vi "_iWorx - Pulse.vi"() -> ()   [LabVIEW 2012]
uses:
  <vilib>/DAQmx/create/channels.llb/DAQmx Create Channel (AI-Voltage-Basic).vi
  <vilib>/DAQmx/configure/timing.llb/DAQmx Timing (Sample Clock).vi
  <vilib>/DAQmx/read.llb/DAQmx Read (Analog 1D Wfm NChan NSamp).vi
  <vilib>/measure/macond.llb/IIR Filter for 1 Chan.vi
  <vilib>/measure/NI_MAPro.lvlib
panel:
  in  "Stop":bool
  in  "Reset Scale":bool
  in  "Log Info Button":bool
  out "Heart Signal":waveform(dbl)(graph)
  out "Avg Pulse":dbl format="%5.1f BPM"
  out "Inst Pulse":dbl format="%5.1f BPM"
  in  "Threshold":dbl=0.0005 step=0.0001 format="%_3p"
  in  "Calibrate":bool
  out "error out":errorcluster
  in  "Set Up":bool
  in  "Channel":u16(ring) items=["Channel 1", "Channel 2"]
  in  "Pause Button":bool
  in  "Snapshot":bool
  in  "Clear Chart":bool
  in  "Open Log":bool
  in  "Rescale Y":bool
  out "Raw Signal":dbl(knob) scale=-1.0..1.0
  # "iWorx - Pulse - Data Logger"
  # "Sensor Input"
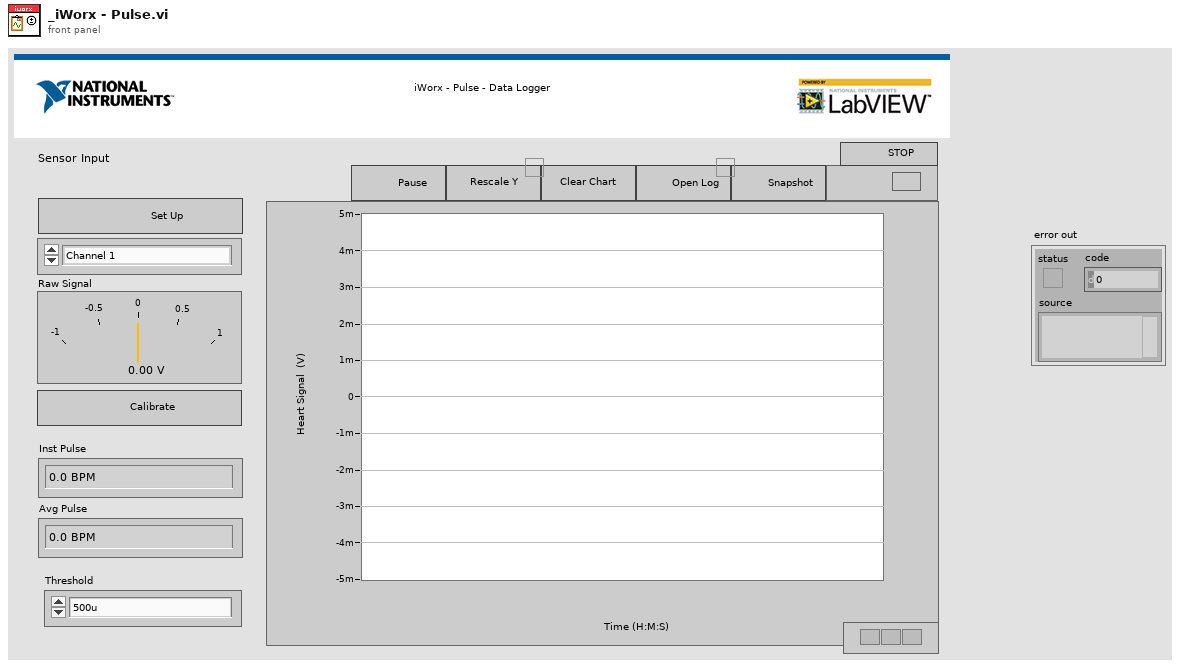
[diagram p1: front panel]
types:
  T1 = cluster{"Topology":enum16{"Off", "Butterworth", "Chebyshev", "Inverse Chebyshev", "Elliptic", "Bessel"}, "Type":enum16{"Lowpass", "Highpass", "Bandpass", "Bandstop"}, "Order":i32, "Lower Fc":dbl, "Upper Fc":dbl, "PB Ripple":dbl, "SB Attenuation":dbl}
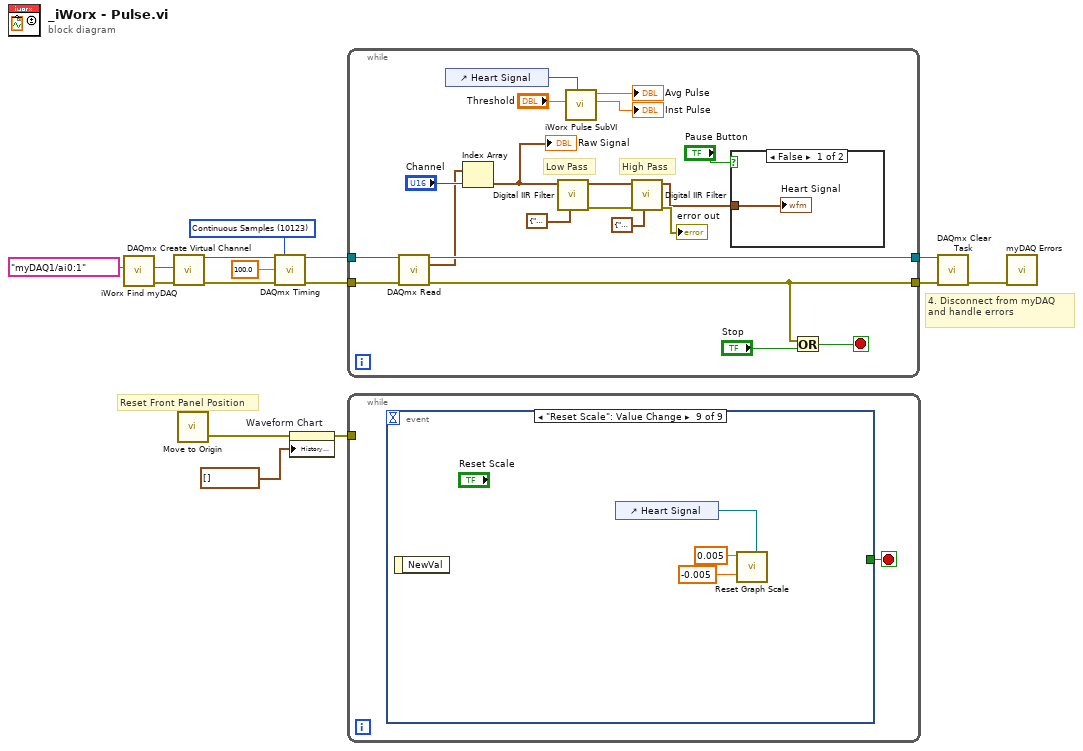
[diagram p0: block diagram]
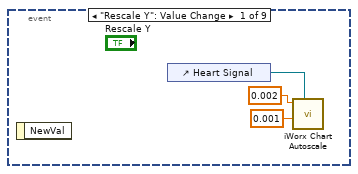
[diagram p2: hidden frame]
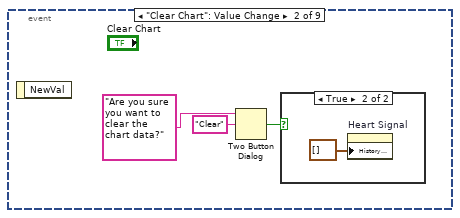
[diagram p3: hidden frame]
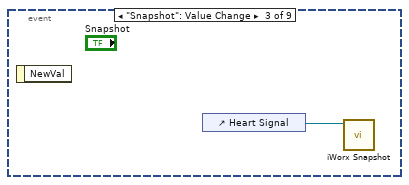
[diagram p5: hidden frame]
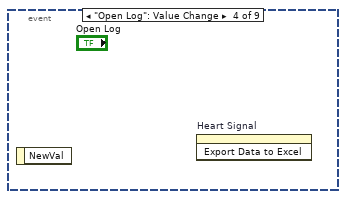
[diagram p6: hidden frame]
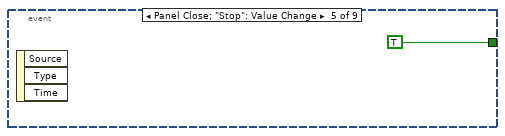
[diagram p7: hidden frame]
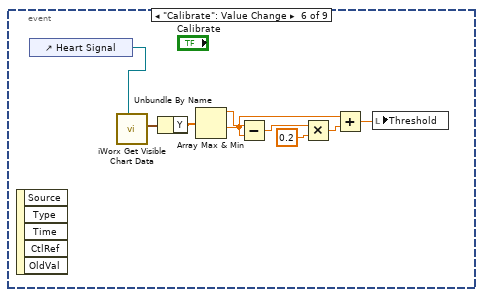
[diagram p8: hidden frame]
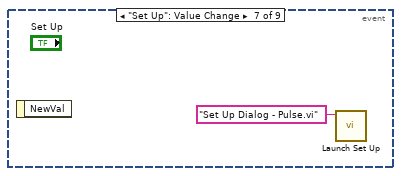
[diagram p9: hidden frame]
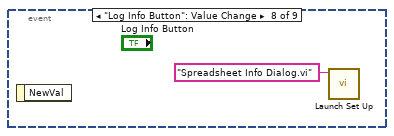
[diagram p10: hidden frame]
diagram:
  w7 = 10123 items=["Finite Samples"=10178, "Continuous Samples"=10123, "Hardware Timed Single Point"=12522] ("sample mode")
  # "4. Disconnect from myDAQ and handle errors"
  # "Reset Front Panel Position"
  n1 = call "iWorx Find myDAQ.vi"("Preferred myDAQ (myDAQ1)"=tag "myDAQ1/ai0:1" ("physical channels")) -> ("Error Out"=w3:errorcluster, "DAQmx Physical Channel"=w4:tag)  [unwired: 6 in, 3 out]
  n2 = call-poly <vilib>:"DAQmx Create Virtual Channel.vi"("physical channels"=w4, "error in"=w3) -> ("task out"=w11:refnum<k21>, "error out"=w10:errorcluster)  [unwired: 12 in]
  n3 = call "Move to Origin.vi"() -> ("Error Out"=w5:errorcluster)  [unwired: 3 in]
  n4 = call-poly <vilib>:"DAQmx Timing.vi"("task/channels in"=w11, "sample mode"=w7, "rate"=100.0, "error in"=w10) -> ("task out"=w8:refnum<k21>, "error out"=w9:errorcluster)  [unwired: 10 in]
  n5 = property on="Waveform Chart" class="WFChart (strict)"(error in=w5, "History Data"=waveform(dbl)[] []) -> (error out=w12:errorcluster)  [unwired: 1 in, 1 out]
  n6 = while {
    tunnel: w8 -> [w35]
    tunnel: [w34] -> w15
    tunnel: w9 -> [w33]
    tunnel: [w31] -> w14
    stop <- w32 stop-if-true
    # "High Pass"
    # "Low Pass"
    n7 = call-poly <vilib>:"DAQmx Read.vi"("task/channels in"=w35, "error in"=w33) -> ("task out"=w34:refnum<k21>, "data"=w28:waveform(dbl)[], "error out"=w31:errorcluster)  [unwired: 11 in]
    n8 = control-ref of="Heart Signal"() -> (w21:refnum<vi>)
    n9 = Index Array(array=w28, index="Channel") -> (element=w19:waveform(dbl))
    "Raw Signal" <- w19
    n10 = call-poly <vilib>:"Digital IIR Filter.vi"("IIR filter specifications"=T1 {"Topology"=enum."Butterworth", "Type"=enum."Lowpass", "Order"=1, "Lower Fc"=0.001, "Upper Fc"=200.0, "PB Ripple"=1.0, "SB Attenuation"=60.0}, "signal in"=w19) -> ("error out"=w25:errorcluster, "signal out"=w22:waveform(dbl))  [unwired: 7 in, 1 out]
    n11 = call "iWorx Pulse SubVI.vi"("Pulse Chart"=w21, "Threshold (.5mV)"="Threshold") -> ("Inst Pulse Rate (BPM)"=→"Inst Pulse":dbl, "Average Pulse Rate (BPM)"=→"Avg Pulse":dbl)  [unwired: 7 in, 1 out]
    n12 = call-poly <vilib>:"Digital IIR Filter.vi"("IIR filter specifications"=T1 {"Topology"=enum."Butterworth", "Type"=enum."Highpass", "Order"=1, "Lower Fc"=1.0, "Upper Fc"=10.0, "PB Ripple"=1.0, "SB Attenuation"=60.0} ("IIR filter specifications 2"), "error in (no error)"=w25, "signal in"=w22) -> ("error out"=→"error out":errorcluster, "signal out"=w24:waveform(dbl))  [unwired: 6 in, 1 out]
    n13 = case shown="False" "Pause Button" {
      tunnel: w24 -> [w36 _]
      frame False {
        "Heart Signal" <- w36
      }
      frame True {
      }
    }
    n14 = Or(x=w31, y="Stop") -> (x .or. y?=w32:bool)
  }
  n15 = while {
    tunnel: w12 -> [_]
    stop <- w37 stop-if-true
    n16 = event shown="[8] \"Reset Scale\": Value Change" {
      selector: _ -> [_ _ _ _ _ _ _ _ _]
      dyn-events: _ -> [_ _ _ _ _ _ _ _ _]
      timeout: _ -> [_ _ _ _ _ _ _ _ _]
      tunnel: [_ _ _ _ TRUE _ _ _ _] -> w37
      event "Rescale Y": Value Change {
        n17 = event-data() -> ()  [unwired: 1 in, 1 out]
        n18 = control-ref of="Heart Signal"() -> (w39:refnum<vi>)
        n19 = call "iWorx Chart Autoscale.vi"("Selection Chart"=w39, "Rounding Multiple (1)"=0.001, "Min Range (1)"=0.002 ("Rounding Multiple (1)")) -> ()  [unwired: 6 in, 3 out]
      }
      event "Clear Chart": Value Change {
        n20 = event-data() -> ()  [unwired: 1 in, 1 out]
        n21 = Two Button Dialog(message="Are you sure you want to clear the chart data?", 2:"Clear" ("T button name (\"OK\")")) -> (T button?=w42:bool)  [unwired: 1 in]
        n22 = case shown="True" w42 {
          frame False {
          }
          frame True {
            n23 = property on="Heart Signal" class="WFChart (strict)"("History Data"=waveform(dbl)[] []) -> ()  [unwired: 2 in, 2 out]
          }
        }
      }
      event "Snapshot": Value Change {
        n24 = event-data() -> ()  [unwired: 1 in, 1 out]
        n25 = control-ref of="Heart Signal"() -> (w45:refnum<vi>)
        n26 = call "iWorx Snapshot.vi"("WaveformChart in"=w45) -> ()  [unwired: 10 in, 1 out]
      }
      event "Open Log": Value Change {
        n27 = event-data() -> ()  [unwired: 1 in, 1 out]
        n28 = invoke on="Heart Signal" class="WFChart (strict)" method="Export Data to Excel"() -> ()  [unwired: 3 in, 3 out]
      }
      event Panel Close; "Stop": Value Change {
        n29 = event-data() -> ()  [unwired: 1 in, 3 out]
      }
      event "Calibrate": Value Change {
        n30 = event-data() -> ()  [unwired: 1 in, 5 out]
        n31 = control-ref of="Heart Signal"() -> (w54:refnum<vi>)
        n32 = call "iWorx Get Visible Chart Data.vi"("Selection Chart"=w54) -> ("waveform out"=w55:waveform(dbl))  [unwired: 8 in, 2 out]
        n33 = Unbundle By Name(w55) -> ("Y"=w48:dbl[])
        n34 = Array Max & Min(array=w48) -> (max value=w49:dbl, min value=w53:dbl)  [unwired: 2 out]
        n35 = Subtract(x=w49, y=w53) -> (x-y=w50:dbl)
        n36 = Multiply(x=w50, y=0.2) -> (x*y=w52:dbl)
        n37 = Add(x=w53, y=w52) -> (x+y=w47:dbl)
        n38 = local write "Threshold"(w47) -> ()
      }
      event "Set Up": Value Change {
        n39 = event-data() -> ()  [unwired: 1 in, 1 out]
        n40 = call "Launch Set Up.vi"("name or relative path"="Set Up Dialog - Pulse.vi") -> ()  [unwired: 9 in, 2 out]
      }
      event "Log Info Button": Value Change {
        n41 = event-data() -> ()  [unwired: 1 in, 1 out]
        n42 = call "Launch Set Up.vi"("name or relative path"="Spreadsheet Info Dialog.vi") -> ()  [unwired: 9 in, 2 out]
      }
      event "Reset Scale": Value Change {
        n43 = event-data() -> ()  [unwired: 1 in, 1 out]
        n44 = control-ref of="Heart Signal"() -> (w59:refnum<vi>)
        n45 = call "Reset Graph Scale.vi"("WaveformChart in"=w59, "Minimum (0)"=-0.005, "Maximum (100)"=0.005) -> ()  [unwired: 9 in]
      }
    }
  }
  n46 = call <vilib>:"DAQmx Clear Task.vi"("task in"=w15, "error in"=w14) -> ("error out"=w1:errorcluster)  [unwired: 13 in]
  n47 = call "myDAQ Errors.vi"("error in (no error)"=w1) -> ()  [unwired: 10 in, 1 out]
